vi "analize weight and theta.vi"(10 "relative object data":T1) -> (1 "weight":sgl, 3 "theta":sgl)   [LabVIEW 2009]
uses:
  object relations.ctl
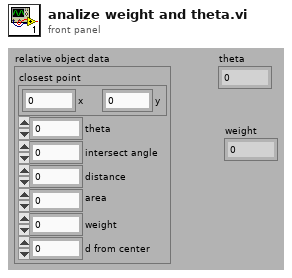
[diagram p1: front panel]
types:
  T1 = typedef "object relations.ctl" = cluster{"closest point":cluster{"x":i16, "y":i16}, "theta":sgl, "intersect angle":sgl, "distance":i16, "area":i16, "weight":sgl, "d from center":i16}
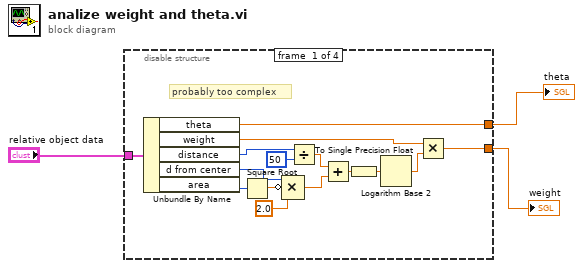
[diagram p0: block diagram]
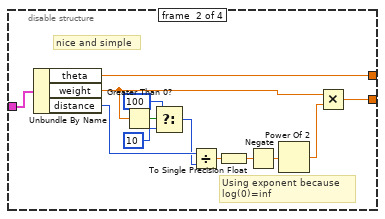
[diagram p2: hidden frame]
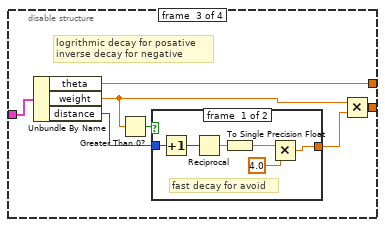
[diagram p3: hidden frame]
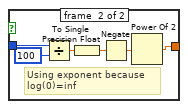
[diagram p4: hidden frame]
diagram:
  n1 = disable-structure shown="Enabled" {
    disable-tunnel: "relative object data" -> [w18 w31 w38 _]
    disable-tunnel: [w6 w29 w36 _] -> w2
    disable-tunnel: [w4 w28 w35 _] -> w1
    frame #0 {
      # "probably too complex"
      n2 = Unbundle By Name(w18) -> ("theta"=w4:sgl, "weight"=w5:sgl, "distance"=w9:i16, "d from center"=w11:i16, "area"=w8:i16)
      n3 = Square Root(x=w8) -> (sqrt(x)=w12:dbl)
      n4 = Compound Arithmetic op=MULTIPLY(w11, invert w12, 2.0 ("value")) -> (w14:dbl)
      n5 = Divide(x=w9, y=i16 50) -> (x/y=w13:dbl)
      n6 = Add(x=w13, y=w14) -> (x+y=w15:dbl)
      n7 = To Single Precision Float(number=w15) -> (single precision float=w16:sgl)
      n8 = Logarithm Base 2(1:w16) -> (0:w7:sgl)
      n9 = Multiply(x=w5, y=w7) -> (x*y=w6:sgl)
    }
    frame #1 {
      # "Using exponent because\nlog(0)=inf"
      # "nice and simple"
      n10 = Unbundle By Name(w31) -> ("theta"=w28:sgl, "weight"=w23:sgl, "distance"=w30:i16)
      n11 = Greater Than 0?(x=w23) -> (x > 0?=w22:bool)
      n12 = Select(t=i16 100 ("y"), s=w22, f=i16 10 ("y")) -> (s? t:f=w21:i16)
      n13 = Divide(x=w30, y=w21) -> (x/y=w27:dbl)
      n14 = To Single Precision Float(number=w27) -> (single precision float=w26:sgl)
      n15 = Negate(x=w26) -> (-x=w25:sgl)
      n16 = Power Of 2(x=w25) -> (2^x=w24:sgl)
      n17 = Multiply(x=w23, y=w24) -> (x*y=w29:sgl)
    }
    frame #2 {
      # "logrithmic decay for posative\ninverse decay for negative"
      n18 = Unbundle By Name(w38) -> ("theta"=w35:sgl, "weight"=w34:sgl, "distance"=w37:i16)
      n19 = Greater Than 0?(x=w34) -> (x > 0?=w32:bool)
      n20 = case shown="False" w32 {
        tunnel: w37 -> [w44 w50]
        tunnel: [w40 w46] -> w33
        frame #0 {
          # "fast decay for avoid"
          n21 = Increment(x=w44) -> (x+1=w43:i16)
          n22 = Reciprocal(x=w43) -> (1/x=w42:dbl)
          n23 = To Single Precision Float(number=w42) -> (single precision float=w41:sgl)
          n24 = Multiply(x=w41, y=sgl 4.0) -> (x*y=w40:sgl)
        }
        frame #1 {
          # "Using exponent because\nlog(0)=inf"
          n25 = Divide(x=w50, y=i16 100) -> (x/y=w49:dbl)
          n26 = To Single Precision Float(number=w49) -> (single precision float=w48:sgl)
          n27 = Negate(x=w48) -> (-x=w47:sgl)
          n28 = Power Of 2(x=w47) -> (2^x=w46:sgl)
        }
      }
      n29 = Multiply(x=w34, y=w33) -> (x*y=w36:sgl)
    }
    frame #3 {
    }
  }
  "weight" <- w2
  "theta" <- w1
